vi "EditValue.vi"(8 "error in (no error)":errorcluster, 10 "Bounds":T1, 11 "DatagridElement in":refnum<class "DatagridElement.lvclass">) -> (0 "error out":errorcluster, 1 "Tabbed out?":bool, 2 "Value changed?":bool, 3 "DatagridElement out":refnum<class "DatagridElement.lvclass">)   [LabVIEW 2018, in "D Datagrid Library.lvlib" / "DatagridElement.lvclass"]
uses:
  DatagridElement.lvclass
  <vilib>/Utility/miscctls.llb/LVRectTypeDef.ctl
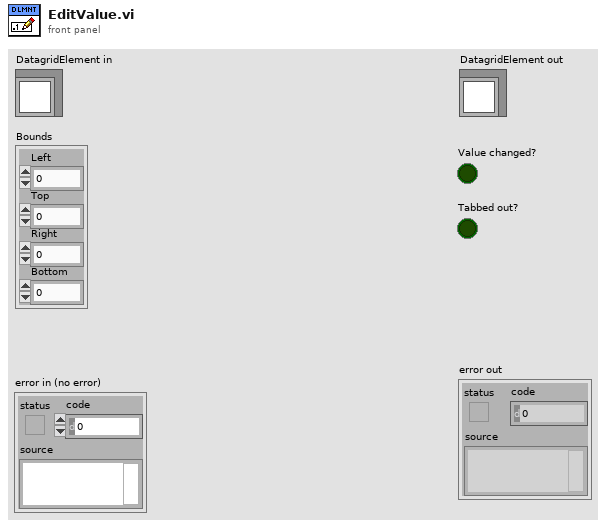
[diagram p1: front panel]
types:
  T1 = typedef "LVRectTypeDef.ctl" = cluster{"Left":i16, "Top":i16, "Right":i16, "Bottom":i16}
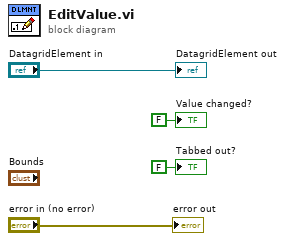
[diagram p0: block diagram]
diagram:
  "error out" <- "error in (no error)"
  "DatagridElement out" <- "DatagridElement in"
  "Value changed?" <- FALSE ("Generate newval event?")
  "Tabbed out?" <- FALSE ("Tabbed out?")
